vi "HFRR ADV v017 new software.vi"() -> ()   [LabVIEW 2025] (continued)
        n325 = Unbundle By Name("Password 3") -> ("Service Password"=w415:string)
        n326 = call <vilib>:"Trim Whitespace.vi"("string"=w415) -> ("trimmed string"=w413:string)  [unwired: 1 in]
        n327 = Equal?(x=w413, y="Service@123") -> (x = y?=w414:bool)
        n328 = case shown="False" w414 {
          selector: w414 -> [w419 w421]
          frame False {
            n329 = local write "Service Password enable"(w419) -> ()
            n330 = property on="Service Password Log" class="Str"("Visible"=TRUE) -> ()  [unwired: 2 in, 2 out]
            n331 = property on="Tab Control 5" class="TabCtl (strict)"("Tabs Visible?"=TRUE ("Page Labels Display Visible?")) -> ()  [unwired: 2 in, 2 out]
          }
          frame True {
            n332 = property on="Service Password Log" class="Str"("Visible"=FALSE) -> ()  [unwired: 2 in, 2 out]
            "Service Password enable" <- w421
          }
        }
      }
      event "Sign In": Value Change {
        w423 = FALSE ("Visible")
        n333 = event-data() -> ()  [unwired: 1 in, 6 out]
        n334 = property on="About" class="Clust (strict)"("Visible"=w423) -> ()  [unwired: 2 in, 2 out]
        n335 = property on="Password 3" class="Clust (strict)"("Visible"=w423) -> ()  [unwired: 2 in, 2 out]
        n336 = property on="Service Password Log" class="Str"("Visible"=FALSE) -> ()  [unwired: 2 in, 2 out]
      }
      event "Info": Value Change {
        n337 = event-data() -> ()  [unwired: 1 in, 6 out]
        n338 = local read "Info"() -> (w425:bool)
        n339 = case shown="False" w425 {
          frame False {
            n340 = property on="About" class="Clust (strict)"("Visible"=FALSE) -> ()  [unwired: 2 in, 2 out]
          }
          frame True {
            n341 = property on="About" class="Clust (strict)"("Visible"=TRUE) -> ()  [unwired: 2 in, 2 out]
          }
        }
      }
      event "Calibration": Value Change {
        n342 = event-data() -> ()  [unwired: 1 in, 6 out]
        n343 = local read "Calibration"() -> (w429:bool)
        n344 = case shown="False" w429 {
          frame False {
            n345 = property on="Calibration 2" class="TabCtl (strict)"("Visible"=FALSE) -> ()  [unwired: 2 in, 2 out]
            n346 = local write "Cal Password"("" ("Cal Password")) -> ()
          }
          frame True {
            n347 = property on="Calibration 2" class="TabCtl (strict)"("Visible"=TRUE) -> ()  [unwired: 2 in, 2 out]
            n348 = local write "Cal Password"("" ("Cal Password")) -> ()
          }
        }
        n349 = property on="Wrong Password" class="Str"("Visible"=FALSE) -> ()  [unwired: 2 in, 2 out]
      }
      event "Cal Password": Value Change {
        n350 = event-data() -> ()  [unwired: 1 in, 6 out]
        n351 = local read "Cal Password"() -> (w437:string)
        n352 = call <vilib>:"Trim Whitespace.vi"("string"=w437) -> ("trimmed string"=w436:string)  [unwired: 1 in]
        n353 = Equal?(x=w436, y="Cal@321") -> (x = y?=w434:bool)
        n354 = case shown="True" w434 {
          frame False {
            n355 = property on="Wrong Password" class="Str"("Visible"=TRUE) -> ()  [unwired: 2 in, 2 out]
          }
          frame True {
            n356 = property on="Wrong Password" class="Str"("Visible"=FALSE) -> ()  [unwired: 2 in, 2 out]
            n357 = local write "Main Tab"(T2."About" ("Main Tab")) -> ()
            n358 = local write "Cal Password"("" ("Cal Password")) -> ()
            n359 = local write "Main Dashboard Buttons"(T1."About" ("Main Dashboard Buttons")) -> ()
            n360 = local write "Tab Control 5"(T12."Temperature Calibration" ("Tab Control 5")) -> ()
            n361 = property on="Calibration 2" class="TabCtl (strict)"("Visible"=FALSE) -> ()  [unwired: 2 in, 2 out]
            n362 = property on="Tab Control 5" class="TabCtl (strict)"("Tabs Visible?"=FALSE ("Page Labels Display Visible?")) -> ()  [unwired: 2 in, 2 out]
            n363 = local write "Calibration"(FALSE ("Calibration")) -> ()
          }
        }
      }
      event "Calibration Selection": Value Change {
        n364 = event-data() -> ()  [unwired: 1 in, 6 out]
        n365 = local read "Calibration Selection"() -> (w448:T8)
        n366 = case shown="\"Stroke Calibration\"" w448 {
          tunnel: [T7."Stroke" ("Main Calibration Tab") T7."Friction" ("Main Calibration Tab") T7."Main" ("Main Calibration Tab") T7."Temperature" ("Main Calibration Tab")] -> w447
          frame "Stroke Calibration" {
          }
          frame "Friction Force Calibration" {
          }
          frame Default {
          }
          frame "Temperature Calibration" {
          }
        }
        n367 = local write "Main Calibration Tab"(w447) -> ()
      }
      event "Back Stroke": Value Change {
        n368 = event-data() -> ()  [unwired: 1 in, 6 out]
        n369 = local write "Main Stroke Tab"(T9."Step 1" ("Main Stroke Tab")) -> ()
        n370 = local write "Main Calibration Tab"(T7."Main" ("Main Calibration Tab")) -> ()
        n371 = local write "Back Stroke"(FALSE ("Back Stroke")) -> ()
      }
      event "Step 2 Back": Value Change {
        n372 = event-data() -> ()  [unwired: 1 in, 6 out]
        n373 = local write "Main Stroke Tab"(T9."Step 1" ("Main Stroke Tab")) -> ()
        n374 = local write "Step 2 Back"(FALSE ("Back Stroke")) -> ()
      }
      event "Step 3 Back": Value Change {
        n375 = event-data() -> ()  [unwired: 1 in, 6 out]
        n376 = local write "Main Stroke Tab"(T9."Step 2" ("Main Stroke Tab")) -> ()
        n377 = local write "Step 3 Back"(FALSE ("Back Stroke")) -> ()
      }
      event "Step 4 Back": Value Change {
        n378 = event-data() -> ()  [unwired: 1 in, 6 out]
        n379 = local write "Main Stroke Tab"(T9."Step 3" ("Main Stroke Tab")) -> ()
        n380 = local write "Step 4 Back"(FALSE ("Back Stroke")) -> ()
      }
      event "Step 5 Back": Value Change {
        n381 = event-data() -> ()  [unwired: 1 in, 6 out]
        n382 = local write "Main Stroke Tab"(T9."Step 4" ("Main Stroke Tab")) -> ()
        n383 = local write "Step 5 Back"(FALSE ("Back Stroke")) -> ()
      }
      event "Step 6 Back": Value Change {
        n384 = event-data() -> ()  [unwired: 1 in, 6 out]
        n385 = local write "Main Stroke Tab"(T9."Step 5" ("Main Stroke Tab")) -> ()
        n386 = local write "Step 6 Back"(FALSE ("Back Stroke")) -> ()
      }
      event "Back Stroke step 7": Value Change {
        n387 = event-data() -> ()  [unwired: 1 in, 6 out]
        n388 = local write "Main Stroke Tab"(T9."Step 6" ("Main Stroke Tab")) -> ()
        n389 = local write "Back Stroke step 7"(FALSE ("Back Stroke")) -> ()
      }
      event "Back Stroke step 8": Value Change {
        n390 = event-data() -> ()  [unwired: 1 in, 6 out]
        n391 = local write "Main Stroke Tab"(T9."Step 7" ("Main Stroke Tab")) -> ()
        n392 = local write "Back Stroke step 8"(FALSE ("Back Stroke")) -> ()
      }
      event "Back Stroke 8": Value Change {
        n393 = event-data() -> ()  [unwired: 1 in, 6 out]
        n394 = local write "MOVE CARRIAGE TO"(0.2 ("MOVE CARRIAGE TO")) -> ()
        n395 = local write "Main Stroke Tab"(T9."Step 1" ("Main Stroke Tab")) -> ()
        n396 = local write "Back Stroke 8"(FALSE ("Back Stroke 8")) -> ()
      }
      event "Continue Stroke": Value Change {
        n397 = event-data() -> ()  [unwired: 1 in, 6 out]
        n398 = local write "Main Stroke Tab"(T9."Step 2" ("Main Stroke Tab")) -> ()
        n399 = local write "Continue Stroke"(FALSE ("Continue Stroke")) -> ()
      }
      event "Continue Stroke step 2": Value Change {
        n400 = event-data() -> ()  [unwired: 1 in, 6 out]
        n401 = local write "Main Stroke Tab"(T9."Step 3" ("Main Stroke Tab")) -> ()
        n402 = local write "Continue Stroke step 2"(FALSE ("Continue Stroke")) -> ()
      }
      event "Continue Stroke step 3": Value Change {
        n403 = event-data() -> ()  [unwired: 1 in, 6 out]
        n404 = local write "Main Stroke Tab"(T9."Step 4" ("Main Stroke Tab")) -> ()
        n405 = local write "Continue Stroke step 3"(FALSE ("Continue Stroke")) -> ()
      }
      event "Continue Stroke step 4": Value Change {
        n406 = event-data() -> ()  [unwired: 1 in, 6 out]
        n407 = local write "Main Stroke Tab"(T9."Step 5" ("Main Stroke Tab")) -> ()
        n408 = local write "Continue Stroke step 4"(FALSE ("Continue Stroke")) -> ()
      }
      event "Continue Stroke step 5": Value Change {
        n409 = event-data() -> ()  [unwired: 1 in, 6 out]
        n410 = local write "Main Stroke Tab"(T9."Step 6" ("Main Stroke Tab")) -> ()
        n411 = local write "Continue Stroke step 5"(FALSE ("Continue Stroke")) -> ()
      }
      event "Continue Stroke step 6": Value Change {
        n412 = event-data() -> ()  [unwired: 1 in, 6 out]
        n413 = local write "Main Stroke Tab"(T9."Step 7" ("Main Stroke Tab")) -> ()
        n414 = local write "Continue Stroke step 6"(FALSE ("Continue Stroke")) -> ()
      }
      event "Continue Stroke step 7": Value Change {
        w487 = FALSE ("0.2mm")
        n415 = event-data() -> ()  [unwired: 1 in, 6 out]
        n416 = local write "0.4 mm"(w487) -> ()
        n417 = local write "0.6 mm"(w487) -> ()
        n418 = local write "1.0 mm"(w487) -> ()
        n419 = local write "1.2 mm"(w487) -> ()
        n420 = local write "0.2 2"(w487) -> ()
        n421 = local write "0.4 2"(w487) -> ()
        n422 = local write "0.6 2"(w487) -> ()
        n423 = local write "0.8 2"(w487) -> ()
        n424 = local write "1.0 2"(w487) -> ()
        n425 = local write "1.2"(w487) -> ()
        n426 = local write "0.2mm"(w487) -> ()
        n427 = local write "0.8mm"(w487) -> ()
        n428 = local write "Main Stroke Tab"(T9."Step 8" ("Main Stroke Tab")) -> ()
        n429 = local write "Continue Stroke step 7"(FALSE ("Continue Stroke")) -> ()
        n430 = local write "Stroke Test Complete"(T10."Test Progress" ("Stroke Test Complete")) -> ()
        "Position Measurment Temp" <- 0.0 ("Position Measurment Temp")
        "Calibration Tare" <- TRUE ("Calibration Tare")
        "MOVE CARRIAGE TO" <- 0.2 ("MOVE CARRIAGE TO")
      }
      event "Continue Stroke step 8": Value Change {
        n431 = event-data() -> ()  [unwired: 1 in, 6 out]
        n432 = local read "LVDT STROKE  Calibration"() -> (w492:dbl)
        n433 = local read "Position Measurment Temp"() -> (w493:dbl)
        n434 = case shown="4" w493 {
          selector: w493 -> [w498 w503 w508 w513 w518 w522 w525 w526]
          tunnel: w492 -> [w494 w499 w504 w509 w514 w519 _ _]
          frame 0, Default {
            w496 = TRUE ("0.2mm")
            n435 = Increment(x=w498) -> (x+1=w497:i32)
            n436 = local write "Position Measurment Temp"(w497) -> ()
            n437 = local write "0.2mm"(w496) -> ()
            n438 = local write "0.2 2"(w496) -> ()
            n439 = local write "MOVE CARRIAGE TO"(0.4 ("MOVE CARRIAGE TO")) -> ()
            "Calibration 0.2" <- w494
          }
          frame 1 {
            w501 = TRUE ("0.4 mm")
            n440 = Increment(x=w503) -> (x+1=w502:i32)
            n441 = local write "Calibration 0.4"(w499) -> ()
            n442 = local write "Position Measurment Temp"(w502) -> ()
            n443 = local write "0.4 mm"(w501) -> ()
            n444 = local write "MOVE CARRIAGE TO"(0.6 ("MOVE CARRIAGE TO")) -> ()
            n445 = local write "0.4 2"(w501) -> ()
          }
          frame 2 {
            w506 = TRUE ("0.6 mm")
            n446 = Increment(x=w508) -> (x+1=w507:i32)
            n447 = local write "Calibration 0.6"(w504) -> ()
            n448 = local write "Position Measurment Temp"(w507) -> ()
            n449 = local write "0.6 2"(w506) -> ()
            n450 = local write "0.6 mm"(w506) -> ()
            n451 = local write "MOVE CARRIAGE TO"(0.8 ("MOVE CARRIAGE TO")) -> ()
          }
          frame 3 {
            w510 = TRUE ("0.6 mm")
            n452 = Increment(x=w513) -> (x+1=w512:i32)
            n453 = local write "Position Measurment Temp"(w512) -> ()
            n454 = local write "MOVE CARRIAGE TO"(1.0 ("MOVE CARRIAGE TO")) -> ()
            n455 = local write "0.8mm"(w510) -> ()
            n456 = local write "0.8 2"(w510) -> ()
            "Calibration 0.8" <- w509
          }
          frame 4 {
            w515 = TRUE ("0.6 mm")
            n457 = Increment(x=w518) -> (x+1=w517:i32)
            n458 = local write "Position Measurment Temp"(w517) -> ()
            n459 = local write "MOVE CARRIAGE TO"(1.2 ("MOVE CARRIAGE TO")) -> ()
            n460 = local write "1.0 mm"(w515) -> ()
            n461 = local write "1.0 2"(w515) -> ()
            "Calibration 1.0" <- w514
          }
          frame 5 {
            w520 = TRUE ("0.6 mm")
            n462 = Increment(x=w522) -> (x+1=w521:i32)
            n463 = local write "Position Measurment Temp"(w521) -> ()
            n464 = local write "1.2 mm"(w520) -> ()
            n465 = local write "1.2"(w520) -> ()
            "Calibration 1.2" <- w519
          }
          frame 6 {
            n466 = Increment(x=w525) -> (x+1=w524:i32)
            n467 = local write "Position Measurment Temp"(w524) -> ()
            n468 = local write "Stroke Test Complete"(T10."Stroke Points Completed" ("Stroke Test Complete")) -> ()
          }
          frame 7 {
            n469 = stacked-sequence {
              tunnel: w526 -> [w527 _ _]
              frame #0 {
                n470 = Increment(x=w527) -> (x+1=w528:i32)
                n471 = local write "Main Stroke Tab"(T9."Step 9" ("Main Stroke Tab")) -> ()
                n472 = local write "Position Measurment Temp"(w528) -> ()
                n473 = Insert Into Array(array=dbl[] [], new element #1=0.2 ("new element/subarray"), new element #2=0.4 ("new element/subarray"), new element #3=0.6 ("new element/subarray"), new element #4=0.8 ("new element/subarray"), new element #5=1.0 ("new element/subarray"), new element #6=1.2 ("new element/subarray")) -> (→"1D stroke":dbl[])  [unwired: 1 in]
                n474 = local read "Calibration 0.2"() -> (w535:dbl)
                n475 = local read "Calibration 0.4"() -> (w534:dbl)
                n476 = local read "Calibration 0.6"() -> (w533:dbl)
                n477 = local read "Calibration 0.8"() -> (w532:dbl)
                n478 = local read "Calibration 1.0"() -> (w531:dbl)
                n479 = local read "Calibration 1.2"() -> (w530:dbl)
                n480 = Insert Into Array(array=dbl[] [], new element #1=w535, new element #2=w534, new element #3=w533, new element #4=w532, new element #5=w531, new element #6=w530) -> (→"Calibrated Voltage Value":dbl[])  [unwired: 1 in]
              }
              frame #1 {
                n481 = local read "Calibrated Voltage Value"() -> (w547:dbl[])
                n482 = local read "1D stroke"() -> (w548:dbl[])
                n483 = for {
                  tunnel: [w551] -> w546 mode=indexing
                  tunnel: w548 -> [w550] mode=indexing
                  tunnel: w547 -> [w549] mode=indexing
                  n484 = formula code="if (stroke == 0.2) {\n    status = (voltage >= 0.0961 && voltage <= 0.4961) ? 1 : 0;\n} else if (stroke == 0.4) {\n    status = (voltage >= 0.3425 && voltage <= 0.7425) ? 1 : 0;\n} else if (stroke == 0.6) {\n    status = (voltage >= 0.5370 && voltage <= 0.9370) ? 1 : 0;\n} else if (stroke == 0.8) {\n    status = (voltage >= 0.6640 && voltage <= 1.0640) ? 1 : 0;\n} else if (stroke == 1.0) {\n    status = (voltage >= 0.9000 && voltage <= 1.1000) ? 1 : 0;\n} else if (stroke == 1.2) {\n    status = (voltage >= 0.9278 && voltage <= 1.3278) ? 1 : 0;\n} else {\n    status = 0; // Fails if an invalid stroke value is supplied\n}"("stroke"=w550, "voltage"=w549) -> ("status"=w551:dbl)
                }
                "Status" <- w546
              }
              frame #2 {
                w558 = 1.0
                n485 = local read "Status"() -> (w565:dbl[])
                n486 = Index Array(array=w565) -> (element #1=w564:dbl, element #2=w563:dbl, element #3=w562:dbl, element #4=w561:dbl, element #5=w560:dbl, element #6=w559:dbl)  [unwired: 6 in]
                n487 = Equal?(x=w563, y=w558) -> (x = y?=w556:bool)
                n488 = Equal?(x=w562, y=w558) -> (x = y?=w555:bool)
                n489 = Equal?(x=w561, y=w558) -> (x = y?=w554:bool)
                n490 = Equal?(x=w560, y=w558) -> (x = y?=w553:bool)
                n491 = Equal?(x=w559, y=w558) -> (x = y?=w552:bool)
                n492 = Equal?(x=w564, y=w558) -> (x = y?=w557:bool)
                n493 = case shown="True" w557 {
                  selector: w557 -> [w576 w577]
                  frame True {
                    n494 = local write "Point 1 - 0.2 mm"(w576) -> ()
                    n495 = property on="Point 1 - 0.2 mm" class="Bool"("Caption.Visible"=w576) -> ()  [unwired: 2 in, 2 out]
                  }
                  frame False {
                    n496 = local write "Point 1 - 0.2 mm"(w577) -> ()
                    n497 = property on="Point 1 - 0.2 mm" class="Bool"("Caption.Visible"=w577) -> ()  [unwired: 2 in, 2 out]
                  }
                }
                n498 = case shown="True" w556 {
                  selector: w556 -> [w574 w575]
                  frame True {
                    n499 = local write "Point 2 - 0.4 mm"(w574) -> ()
                    n500 = property on="Point 2 - 0.4 mm" class="Bool"("Caption.Visible"=w574) -> ()  [unwired: 2 in, 2 out]
                  }
                  frame False {
                    n501 = local write "Point 2 - 0.4 mm"(w575) -> ()
                    n502 = property on="Point 2 - 0.4 mm" class="Bool"("Caption.Visible"=w575) -> ()  [unwired: 2 in, 2 out]
                  }
                }
                n503 = case shown="True" w553 {
                  selector: w553 -> [w568 w569]
                  frame True {
                    n504 = local write "Point 5 - 1.0 mm"(w568) -> ()
                    n505 = property on="Point 5 - 1.0 mm" class="Bool"("Caption.Visible"=w568) -> ()  [unwired: 2 in, 2 out]
                  }
                  frame False {
                    n506 = local write "Point 5 - 1.0 mm"(w569) -> ()
                    n507 = property on="Point 5 - 1.0 mm" class="Bool"("Caption.Visible"=w569) -> ()  [unwired: 2 in, 2 out]
                  }
                }
                n508 = case shown="True" w555 {
                  selector: w555 -> [w572 w573]
                  frame True {
                    n509 = local write "Point 3 - 0.6 mm"(w572) -> ()
                    n510 = property on="Point 3 - 0.6 mm" class="Bool"("Caption.Visible"=w572) -> ()  [unwired: 2 in, 2 out]
                  }
                  frame False {
                    n511 = local write "Point 3 - 0.6 mm"(w573) -> ()
                    n512 = property on="Point 3 - 0.6 mm" class="Bool"("Caption.Visible"=w573) -> ()  [unwired: 2 in, 2 out]
                  }
                }
                n513 = case shown="True" w554 {
                  selector: w554 -> [w570 w571]
                  frame True {
                    n514 = local write "Point 4 - 0.8 mm"(w570) -> ()
                    n515 = property on="Point 4 - 0.8 mm" class="Bool"("Caption.Visible"=w570) -> ()  [unwired: 2 in, 2 out]
                  }
                  frame False {
                    n516 = local write "Point 4 - 0.8 mm"(w571) -> ()
                    n517 = property on="Point 4 - 0.8 mm" class="Bool"("Caption.Visible"=w571) -> ()  [unwired: 2 in, 2 out]
                  }
                }
                n518 = case shown="True" w552 {
                  selector: w552 -> [w566 w567]
                  frame True {
                    n519 = local write "Point 6 - 1.2 mm"(w566) -> ()
                    n520 = property on="Point 6 - 1.2 mm" class="Bool"("Caption.Visible"=w566) -> ()  [unwired: 2 in, 2 out]
                  }
                  frame False {
                    n521 = local write "Point 6 - 1.2 mm"(w567) -> ()
                    n522 = property on="Point 6 - 1.2 mm" class="Bool"("Caption.Visible"=w567) -> ()  [unwired: 2 in, 2 out]
                  }
                }
              }
            }
          }
        }
      }
      event "TEMPERATURE STEP Back 1", "TEMPERATURE STEP Back air Temp": Value Change {
        n523 = event-data() -> ()  [unwired: 1 in, 6 out]
        n524 = stacked-sequence {
          frame #0 {
            n525 = local write "Main Calibration Tab"(T7."Main" ("Main Calibration Tab")) -> ()
          }
          frame #1 {
            n526 = Wait (ms)(milliseconds to wait=u32 1000) -> ()  [unwired: 1 out]
          }
          frame #2 {
            n527 = local write "Command"("CAL;END" ("Command")) -> ()
          }
          frame #3 {
            n528 = Wait (ms)(milliseconds to wait=u32 2000) -> ()  [unwired: 1 out]
          }
          frame #4 {
            n529 = local write "Command"("CAL;END" ("Command")) -> ()
          }
        }
      }
      event "Temperature Continue Step 1": Value Change {
        n530 = event-data() -> ()  [unwired: 1 in, 6 out]
        n531 = stacked-sequence {
          frame #0 {
            n532 = Wait (ms)(milliseconds to wait=u32 1500) -> ()  [unwired: 1 out]
          }
          frame #1 {
            n533 = local write "Command"("CAL;START" ("Command")) -> ()
          }
          frame #2 {
            n534 = Wait (ms)(milliseconds to wait=u32 1500) -> ()  [unwired: 1 out]
          }
          frame #3 {
            n535 = local write "Command"("CAL;START" ("Command")) -> ()
          }
          frame #4 {
            n536 = Wait (ms)(milliseconds to wait=u32 2000) -> ()  [unwired: 1 out]
          }
          frame #5 {
          }
          frame #6 {
            n537 = Wait (ms)(milliseconds to wait=u32 2000) -> ()  [unwired: 1 out]
          }
          frame #7 {
            # "CAL;A1;<true_T>"
            n538 = local write "Command"("CAL;A1;0" ("Command")) -> ()
          }
          frame #8 {
            n539 = local write "Tab Control 4"(T11."Step 2" ("Tab Control 4")) -> ()
          }
        }
      }
      event "Temperature Continue Step air Step 1": Value Change {
        n540 = event-data() -> ()  [unwired: 1 in, 6 out]
        n541 = stacked-sequence {
          frame #0 {
            n542 = Wait (ms)(milliseconds to wait=u32 1500) -> ()  [unwired: 1 out]
          }
          frame #1 {
            n543 = local write "Command"("CAL;START" ("Command")) -> ()
          }
          frame #2 {
            n544 = local write "Tab Control 4"(T11."Air Step 2" ("Tab Control 4")) -> ()
            n545 = Wait (ms)(milliseconds to wait=u32 1500) -> ()  [unwired: 1 out]
          }
          frame #3 {
            n546 = local write "Command"("CAL;START" ("Command")) -> ()
          }
          frame #4 {
            n547 = Wait (ms)(milliseconds to wait=u32 2000) -> ()  [unwired: 1 out]
          }
          frame #5 {
            # "CAL;A1;<true_T>"
            n548 = local write "Command"("CAL;A2;0" ("Command")) -> ()
          }
          frame #6 {
            n549 = Wait (ms)(milliseconds to wait=u32 2000) -> ()  [unwired: 1 out]
          }
          frame #7 {
            # "CAL;A1;<true_T>"
            n550 = local write "Command"("CAL;A1;0" ("Command")) -> ()
          }
        }
      }
      event "Temperature Selection": Value Change {
        n551 = event-data() -> ()  [unwired: 1 in, 6 out]
        n552 = local read "Temperature Selection"() -> (w600:enum32{"Air Temperature", "Sample Temperature"})
        n553 = case shown="\"Sample Temperature\"" w600 {
          frame "Air Temperature", Default {
            n554 = local write "Tab Control 4"(T11."Air Step 1" ("Tab Control 4")) -> ()
          }
          frame "Sample Temperature" {
            n555 = local write "Tab Control 4"(T11."Step 1" ("Tab Control 4")) -> ()
          }
        }
      }
      event "Temperature Continue Step 2": Value Change {
        n556 = event-data() -> ()  [unwired: 1 in, 6 out]
        n557 = stacked-sequence {
          frame #0 {
            n558 = stacked-sequence {
              frame #0 {
                n559 = Wait (ms)(milliseconds to wait=u32 1500) -> ()  [unwired: 1 out]
              }
              frame #1 {
                # "CAL;A1;<true_T>"
                n560 = local write "Command"("CAL;A1;0" ("Command")) -> ()
              }
              frame #2 {
                n561 = Wait (ms)(milliseconds to wait=u32 1500) -> ()  [unwired: 1 out]
              }
              frame #3 {
                # "CAL;A1;<true_T>"
                n562 = local write "Command"("CAL;A1;0" ("Command")) -> ()
              }
              frame #4 {
              }
            }
          }
          frame #1 {
            n563 = local write "Tab Control 4"(T11."Step 3" ("Tab Control 4")) -> ()
          }
        }
      }
      event "Temperature Continue Step 3": Value Change {
        n564 = event-data() -> ()  [unwired: 1 in, 6 out]
        n565 = stacked-sequence {
          frame #0 {
            n566 = stacked-sequence {
              frame #0 {
                n567 = Wait (ms)(milliseconds to wait=u32 1500) -> ()  [unwired: 1 out]
              }
              frame #1 {
              }
              frame #2 {
              }
              frame #3 {
                # "CAL;A1;<true_T>"
                n568 = local write "Command"("CAL;A1;60" ("Command")) -> ()
              }
              frame #4 {
                n569 = Wait (ms)(milliseconds to wait=u32 2000) -> ()  [unwired: 1 out]
              }
              frame #5 {
                # "CAL;A1;<true_T>"
                n570 = local write "Command"("CAL;A1;60" ("Command")) -> ()
              }
            }
          }
          frame #1 {
            n571 = Wait (ms)(milliseconds to wait=u32 1000) -> ()  [unwired: 1 out]
          }
          frame #2 {
            n572 = local write "Command"("CAL;SAVE" ("Command")) -> ()
          }
          frame #3 {
            n573 = Wait (ms)(milliseconds to wait=u32 1000) -> ()  [unwired: 1 out]
          }
          frame #4 {
            n574 = local write "Command"("CAL;SAVE" ("Command")) -> ()
          }
          frame #5 {
            n575 = Wait (ms)(milliseconds to wait=u32 1000) -> ()  [unwired: 1 out]
          }
          frame #6 {
            # "CAL;END"
            n576 = local write "Command"("CAL;END" ("Command")) -> ()
          }
          frame #7 {
            n577 = Wait (ms)(milliseconds to wait=u32 1000) -> ()  [unwired: 1 out]
          }
          frame #8 {
            # "CAL;END"
            n578 = local write "Command"("CAL;END" ("Command")) -> ()
          }
          frame #9 {
            n579 = local write "Main Calibration Tab"(T7."Temperature" ("Main Calibration Tab")) -> ()
            n580 = local write "Tab Control 4"(T11."Main" ("Tab Control 4")) -> ()
          }
        }
      }
      event "Back Stroke step main temperature": Value Change {
        n581 = event-data() -> ()  [unwired: 1 in, 6 out]
        n582 = stacked-sequence {
          frame #0 {
            n583 = Wait (ms)(milliseconds to wait=u32 1000) -> ()  [unwired: 1 out]
          }
          frame #1 {
            # "CAL;END"
            n584 = local write "Command"("CAL;END" ("Command")) -> ()
          }
          frame #2 {
            n585 = Wait (ms)(milliseconds to wait=u32 1000) -> ()  [unwired: 1 out]
          }
          frame #3 {
            # "CAL;END"
            n586 = local write "Command"("CAL;END" ("Command")) -> ()
          }
          frame #4 {
            n587 = local write "Main Calibration Tab"(T7."Temperature" ("Main Calibration Tab")) -> ()
            n588 = local write "Tab Control 4"(T11."Main" ("Tab Control 4")) -> ()
          }
        }
      }
      event "Quit": Value Change {
        n589 = event-data() -> ()  [unwired: 1 in, 6 out]
      }
    }
    n590 = Wait (ms)(milliseconds to wait=u32 100) -> ()  [unwired: 1 out]
  }
  n591 = while {
    stop <- w632 stop-if-true
    n592 = local read "Ambient Temperature"() -> (w630:dbl)
    n593 = local read "Sample Temperature"() -> (w629:dbl)
    n594 = local write "Temperature — Live (Set A: 60 °C)"(w629) -> ()
    n595 = local write "Temperature — Live (Set A: 60 °C)"(w629) -> ()
    n596 = local write "Temperature — Live (Set A: 0 °C)"(w630) -> ()
    n597 = local write "Sensor value"(w630) -> ()
    n598 = local write "Sensor value"(w629) -> ()
    n599 = local write "Temperature — Live (Set A: 60 °C)"(w630) -> ()
    n600 = local write "Sensor value"(w629) -> ()
    n601 = local write "Sensor value"(w630) -> ()
    n602 = Wait (ms)(milliseconds to wait=u32 200) -> ()  [unwired: 1 out]
    n603 = local read "Quit"() -> (w632:bool)
  }
  n604 = while {
    shift-right: [w634] -> _
    shift-left: "Enum - Selector" -> [w635]
    stop <- w636 stop-if-true
    # "Auto Start Logic Loop"
    n605 = case shown="\"Maintain Stage\"" w635 {
      tunnel: [w639 w645 w672 w704 w734 Auto_Start_enum."Exit" ("Enum - Selector") Auto_Start_enum."Init" ("Enum - Selector")] -> w634
      frame "Init", Default {
        n606 = local read "Auto Start Test"() -> (w638:bool)
        n607 = Select(t=Auto_Start_enum."Humidity & Temperature On" ("Enum - Selector"), s=w638, f=Auto_Start_enum."Init") -> (s? t:f=w639:T15)
      }
      frame "Humidity & Temperature On" {
        n608 = stacked-sequence {
          tunnel: [_ _ _ _ _ _ Auto_Start_enum."Reach point" ("Enum - Selector")] -> w642
          frame #0 {
            w647 = T19."Disabled and Grayed Out" ("Disabled")
            w648 = TRUE ("Heater Button")
            n609 = property on="Humidity" class="Bool (strict)"("DisabledEnum"=w647) -> ()  [unwired: 2 in, 2 out]
            n610 = property on="Heater Button" class="Bool (strict)"("DisabledEnum"=w647) -> ()  [unwired: 2 in, 2 out]
            n611 = local write "Heater Button"(w648) -> ()
            n612 = local write "Humidity"(w648) -> ()
            n613 = property on="Heater Button" class="Bool (strict)"("Val(Sgnl)"=TRUE ("Value (Signaling)")) -> ()  [unwired: 2 in, 2 out]
          }
          frame #1 {
            n614 = Wait (ms)(milliseconds to wait=u32 3000) -> ()  [unwired: 1 out]
          }
          frame #2 {
            n615 = local read "Set Temp"() -> (w654:dbl)
            n616 = Number To Fractional String(number=w654, precision (6)=i16 2) -> (F-format string=w651:string)  [unwired: 2 in]
            n617 = Concatenate Strings("ST;" ("Command"), w651) -> (w652:string)
            n618 = local write "Command"(w652) -> ()
          }
          frame #3 {
            n619 = Wait (ms)(milliseconds to wait=u32 1500) -> ()  [unwired: 1 out]
          }
          frame #4 {
            (unwired) i16 2 ("precision (6)")
            n620 = local read "Set Rh"() -> (w657:dbl)
            n621 = Number To Fractional String(number=w657) -> (F-format string=w660:string)  [unwired: 3 in]
            n622 = local read "WriteHumidity"() -> (w658:string[])
            n623 = Concatenate Strings("M;" ("new element/subarray"), w660) -> (w661:string)
            n624 = local write "Command"("HE;1" ("Command")) -> ()
            n625 = Insert Into Array(array=w658, new element=w661) -> (w659:string[])  [unwired: 1 in]
            n626 = local write "WriteHumidity"(w659) -> ()
          }
          frame #5 {
            n627 = Wait (ms)(milliseconds to wait=u32 1500) -> ()  [unwired: 1 out]
          }
          frame #6 {
            w664 = TRUE ("Reach point temp")
            n628 = local write "Reach point Humidity"(w664) -> ()
            n629 = local write "Reach point temp"(w664) -> ()
          }
        }
        n630 = local read "Auto Start Test"() -> (w644:bool)
        n631 = Not(x=w644) -> (.not. x?=w643:bool)
        n632 = Select(t=Auto_Start_enum."close", s=w643, f=w642) -> (s? t:f=w645:T15)
      }
      frame "Reach point" {
        w673 = TRUE ("PAUSE")
        w681 = 1.0 ("y")
        w684 = 1.0 ("y")
        n633 = local read "Set Temp"() -> (w666:dbl)
        n634 = local read "Set Humidity:"() -> (w680:dbl)
        n635 = local read "Humidity ( %RH )"() -> (w685:dbl)
        n636 = Add(x=w666, y=w684) -> (x+y=w683:dbl)
        n637 = Subtract(x=w666, y=w684) -> (x-y=w682:dbl)
        n638 = Add(x=w680, y=w681) -> (x+y=w679:dbl)
        n639 = Subtract(x=w680, y=w681) -> (x-y=w678:dbl)
        n640 = local read "TEMP"() -> (w686:dbl)
        n641 = In Range and Coerce(upper limit=w679, x=w685, lower limit=w678) -> (In Range?=w667:bool)  [unwired: 1 out]
        n642 = In Range and Coerce(upper limit=w683, x=w686, lower limit=w682) -> (In Range?=w668:bool)  [unwired: 1 out]
        n643 = case shown="True" w667 {
          frame False {
          }
          frame True {
            n644 = case shown="True" "Reach point Humidity" {
              selector: "Reach point Humidity" -> [_ w692]
              frame False {
              }
              frame True {
                n645 = local read "EVENT LOG"() -> (w689:string)
                n646 = Not(x=w692) -> (.not. x?=w691:bool)
                n647 = local write "Reach point Humidity"(w691) -> ()
                n648 = call "Event Log.vi"("Content"="Target Humidity reached", "EVENT LOG"=w689) -> ("EVENT LOG"=w690:string)  [unwired: 8 in, 1 out]
                n649 = local write "EVENT LOG"(w690) -> ()
              }
            }
          }
        }
        n650 = case shown="True" w668 {
          frame False {
          }
          frame True {
            n651 = case shown="True" "Reach point temp" {
              selector: "Reach point temp" -> [_ w698]
              frame False {
              }
              frame True {
                n652 = local read "EVENT LOG"() -> (w695:string)
                n653 = Not(x=w698) -> (.not. x?=w697:bool)
                n654 = local write "Reach point temp"(w697) -> ()
                n655 = call "Event Log.vi"("Content"="Target Temperature reached", "EVENT LOG"=w695) -> ("EVENT LOG"=w696:string)  [unwired: 8 in, 1 out]
                n656 = local write "EVENT LOG"(w696) -> ()
              }
            }
          }
        }
        n657 = local read "Auto Start Test"() -> (w671:bool)
        n658 = And(x=w668, y=w667) -> (x .and. y?=w677:bool)
        n659 = Select(t=Auto_Start_enum."Maintain Stage" ("Enum - Selector"), s=w677, f=Auto_Start_enum."Reach point" ("Enum - Selector")) -> (s? t:f=w674:T15)
        n660 = Not(x=w671) -> (.not. x?=w670:bool)
        n661 = Select(t=Auto_Start_enum."close", s=w670, f=w674) -> (s? t:f=w672:T15)
        n662 = call "ELAPSED TIMER VI.vi"("RESET"=w673, "PAUSE"=w673) -> ()  [unwired: 7 in, 3 out]
      }
      frame "Maintain Stage" {
        w713 = 2.0 ("y")
        w712 = 1.0 ("y")
        # "Humidity and  temperatures Set Point  have been reached"
        n663 = local read "Set Temp"() -> (w699:dbl)
        n664 = local read "Set Humidity:"() -> (w716:dbl)
        n665 = local read "Humidity ( %RH )"() -> (w719:dbl)
        n666 = Add(x=w699, y=w712) -> (x+y=w718:dbl)
        n667 = Subtract(x=w699, y=w712) -> (x-y=w717:dbl)
        n668 = local read "TEMP"() -> (w720:dbl)
        n669 = Add(x=w716, y=w713) -> (x+y=w715:dbl)
        n670 = Subtract(x=w716, y=w713) -> (x-y=w714:dbl)
        n671 = In Range and Coerce(upper limit=w718, x=w720, lower limit=w717) -> (In Range?=w711:bool)  [unwired: 1 out]
        n672 = In Range and Coerce(upper limit=w715, x=w719, lower limit=w714) -> (In Range?=w710:bool)  [unwired: 1 out]
        n673 = And(x=w711, y=w710) -> (x .and. y?=w709:bool)
        n674 = Not(x=w709) -> (.not. x?=w708:bool)
        n675 = call "ELAPSED TIMER VI.vi"("TARGET"=60.0, "RESET"=w708, "PAUSE"=FALSE) -> ("ELAPSED INDICATION"=w705:bool)  [unwired: 6 in, 2 out]
        n676 = case shown="True" w705 {
          tunnel: w705 -> [_ w723]
          tunnel: [Auto_Start_enum."Maintain Stage" ("Enum - Selector") w722] -> w703
          frame False {
          }
          frame True {
            n677 = stacked-sequence {
              tunnel: w723 -> [_ _ _ _ _]
              tunnel: [_ _ _ _ Auto_Start_enum."Start Stage" ("Enum - Selector")] -> w722
              frame #0 {
                n678 = local read "EVENT LOG"() -> (w725:string)
                n679 = call "Event Log.vi"("Content"="Humidity and temperature set point has stabilized.", "EVENT LOG"=w725) -> ("EVENT LOG"=w726:string)  [unwired: 8 in, 1 out]
                n680 = local write "EVENT LOG"(w726) -> ()
              }
              frame #1 {
                n681 = Wait (ms)(milliseconds to wait=u32 100) -> ()  [unwired: 1 out]
              }
              frame #2 {
                n682 = local read "EVENT LOG"() -> (w729:string)
                n683 = call "Event Log.vi"("Content"="Auto Test Started", "EVENT LOG"=w729) -> ("EVENT LOG"=w730:string)  [unwired: 8 in, 1 out]
                n684 = local write "EVENT LOG"(w730) -> ()
              }
              frame #3 {
                w731 = TRUE ("RUN")
                n685 = local write "RUN"(w731) -> ()
                n686 = property on="Auto Start Temp" class="Bool (strict)"("Val(Sgnl)"=w731) -> ()  [unwired: 2 in, 2 out]
                "Auto Start Temp" <- w731
              }
              frame #4 {
              }
            }
          }
        }
        n687 = local read "Auto Start Test"() -> (w702:bool)
        n688 = Not(x=w702) -> (.not. x?=w701:bool)
        n689 = Select(t=Auto_Start_enum."close", s=w701, f=w703) -> (s? t:f=w704:T15)
      }
      frame "Start Stage" {
        w733 = TRUE ("PAUSE")
        n690 = local read "Auto Start Test"() -> (w738:bool)
        n691 = Not(x=w738) -> (.not. x?=w737:bool)
        n692 = Select(t=Auto_Start_enum."close" ("Enum - Selector"), s=w737, f=Auto_Start_enum."Start Stage" ("Enum - Selector")) -> (s? t:f=w734:T15)
        n693 = call "ELAPSED TIMER VI.vi"("RESET"=w733, "PAUSE"=w733) -> ()  [unwired: 7 in, 3 out]
      }
      frame "close" {
        w740 = FALSE ("Heater Button")
        n694 = local write "RUN"(w740) -> ()
        n695 = local write "Heater Button"(w740) -> ()
        n696 = local write "Humidity"(w740) -> ()
        n697 = local write "Auto Start Test"(w740) -> ()
        n698 = property on="Heater Button" class="Bool (strict)"("Val(Sgnl)"=FALSE ("Value (Signaling)")) -> ()  [unwired: 2 in, 2 out]
      }
      frame "Exit" {
      }
    }
    n699 = Wait (ms)(milliseconds to wait=u32 100) -> ()  [unwired: 1 out]
    n700 = local read "Quit"() -> (w636:bool)
  }
  n701 = property on="Service Password Log" class="Str"("Visible"=w15) -> ()  [unwired: 2 in, 2 out]
  n702 = property on="Password 3" class="Clust (strict)"("Visible"=w15) -> ()  [unwired: 2 in, 2 out]
  n703 = while {
    stop <- w769 stop-if-true
    w752 = errorcluster {"status"=FALSE, "code"=0, "source"=""} ("error in (no error) 3")
    # "this loop is for manual report generation"
    n704 = local read "Confirm Measrurement"() -> (w751:bool)
    n705 = case shown="True" w751 {
      selector: w751 -> [_ w859]
      tunnel: errorcluster {"status"=FALSE, "code"=0, "source"=""} ("error in (no error) 3") -> [_ w860]
      tunnel: [_ w858] -> _
      frame False {
      }
      frame True {
        n706 = stacked-sequence {
          tunnel: w860 -> [_ w893 _]
          tunnel: w859 -> [_ _ w1000]
          tunnel: [_ w881 _] -> w858
          frame #0 {
            n707 = String To Path(string="C:\\LAB-IQ\\Image Calibrate v01.dcf") -> (path=w863:path)
            n708 = Open/Create/Replace File ("Open File")(file path (use dialog)=w863) -> (refnum out=w864:refnum<file>)  [unwired: 5 in, 2 out]
            n709 = for {
              N: 4 -> [_]
              tunnel: w864 -> [w870]
              i -> [w866]
              n710 = Read from Text File ("Read File")(file (use dialog)=w870) -> (text=w871:string)  [unwired: 3 in, 3 out]
              n711 = String Subset(string=w871, offset (0)=6, length (rest)=10 ("length (rest)")) -> (substring=w867:string)
              n712 = Fract/Exp String To Number(string=w867) -> (number=w865:dbl)  [unwired: 3 in, 1 out]
              n713 = case shown="3" w866 {
                tunnel: w865 -> [w872 w873 _ w874 _]
                frame 0 {
                  n714 = local write "5x Gain"(w872) -> ()
                }
                frame 1 {
                  n715 = local write "10x Gain"(w873) -> ()
                }
                frame 2 {
                }
                frame 3 {
                  n716 = local write "100x gain"(w874) -> ()
                }
                frame 4, Default {
                }
              }
            }
          }
          frame #1 {
            n717 = local read "TEST STANDARD"() -> (w876:T3)
            n718 = case shown="\"ISO 12156\"" w876 {
              tunnel: ["ASTM D6079" "ISO 12156"] -> w875
              frame "ASTM D6079", Default {
              }
              frame "ISO 12156" {
              }
            }
            n719 = call "IMAGE ANALYSIS.vi"("Enum"=POST_ANALYSIS_ENUM."GET MEASUREMENTS", "error in"=w893) -> ("error out"=w900:errorcluster)  [unwired: 8 in, 1 out]
            n720 = local read "Magnification :"() -> (w886:string)
            n721 = call "Stall Data Flow.vim"("value in"=w900, "milliseconds to wait"=u32 1000) -> ("value out"=w899:errorcluster)  [unwired: 1 out]
            n722 = local read "Test File List :"() -> (w897:string)
            n723 = case shown="\"10x\"" w886 {
              tunnel: [w936 w937] -> w884
              frame "5x", Default {
                n724 = local read "5x Gain"() -> (w936:dbl)
              }
              frame "10x" {
                # "5x"
                n725 = local read "10x Gain"() -> (w937:dbl)
              }
            }
            n726 = call "IMAGE ANALYSIS.vi"("Enum"=POST_ANALYSIS_ENUM."READ", "error in"=w899) -> ("error out"=w896:errorcluster, "data out"=w887:string)  [unwired: 8 in]
            n727 = Match Pattern(string=w887, regular expression="\"type\": ") -> (after substring=w891:string)  [unwired: 1 in, 3 out]
            n728 = call "IMAGE PATH CREATION PY.vi"("error in (no error)"=w896, "File Name :"=w897) -> ("error out"=w895:errorcluster, "File Path"=w883:path, "File Path String:"=w878:string)  [unwired: 7 in]
            n729 = Match Pattern(string=w891, regular expression=",") -> (before substring=w877:string)  [unwired: 1 in, 3 out]
            n730 = local read "Calibration Tab"() -> (w880:enum32{"Measrument", "Calibrate"})
            n731 = call "Stall Data Flow.vim"("value in"=w895, "milliseconds to wait"=u32 250) -> ("value out"=w879:errorcluster)  [unwired: 1 out]
            n732 = Equal?(x=w877, y="\"rectangle\"") -> (x = y?=w888:bool)
            n733 = case shown="False" w888 {
              tunnel: w887 -> [w942 w997]
              tunnel: w884 -> [_ w988]
              tunnel: cluster{"major":dbl, "minor":dbl, "average":dbl} {"major"=0.0, "minor"=0.0, "average"=0.0} -> [w940 w984]
              tunnel: [w939 w981] -> w882
              tunnel: w877 -> [w941 _]
              tunnel: w884 -> [w938 _]
              frame False {
                n734 = Equal?(x=w941, y="\"line\"") -> (x = y?=w943:bool)
                n735 = case shown="True" w943 {
                  tunnel: w942 -> [_ w958]
                  tunnel: w940 -> [w945 w957]
                  tunnel: [w945 w955] -> w939
                  tunnel: w938 -> [_ w954]
                  frame False {
                  }
                  frame True {
                    w953 = 0.0 ("Major Axis")
                    n736 = Match Pattern(string=w958, regular expression="\"length_px\":") -> (after substring=w956:string)  [unwired: 1 in, 3 out]
                    n737 = property on="Major Axis" class="DigNum (strict)"("Caption.Text"="") -> ()  [unwired: 2 in, 2 out]
                    n738 = property on="Minor Axis" class="DigNum (strict)"("Caption.Text"="") -> ()  [unwired: 2 in, 2 out]
                    n739 = property on="Average" class="DigNum (strict)"("Caption.Text"="Line") -> ()  [unwired: 2 in, 2 out]
                    n740 = Fract/Exp String To Number(string=w956, default (0 dbl)=0.0 ("default (0 DBL)")) -> (number=w952:dbl)  [unwired: 2 in, 1 out]
                    "Pixel Value" <- w952
                    n741 = Multiply(x=w952, y=w954) -> (x*y=w965:dbl)
                    n742 = Multiply(x=w965, y=1000.0) -> (x*y=w948:dbl)
                    n743 = Divide(x=w948, y=1000.0) -> (x/y=w951:dbl)
                    n744 = local write "Measurment (mm)"(w951) -> ()
                    n745 = Bundle By Name(cluster=w957, "average"=w948) -> (w955:cluster{"major":dbl, "minor":dbl, "average":dbl})
                    n746 = Number To Fractional String(number=w948, precision (6)=i16 1) -> (F-format string=w947:string)  [unwired: 2 in]
                    n747 = local write "Minor Axis"(w953) -> ()
                    n748 = local write "Major Axis"(w953) -> ()
                    n749 = Fract/Exp String To Number(string=w947) -> (number=w946:dbl)  [unwired: 3 in, 1 out]
                    n750 = local write "Average"(w946) -> ()
                  }
                }
              }
              frame True {
                w985 = 1000.0 ("y")
                w991 = 0.0 ("default (0 DBL)")
                n751 = Match Pattern(string=w997, regular expression=" \"width_px\":") -> (after substring=w995:string)  [unwired: 1 in, 3 out]
                n752 = Match Pattern(string=w995, regular expression="\"height_px\":") -> (before substring=w993:string, after substring=w992:string)  [unwired: 1 in, 2 out]
                n753 = Fract/Exp String To Number(string=w993, default (0 dbl)=w991) -> (number=w990:dbl)  [unwired: 2 in, 1 out]
                n754 = Fract/Exp String To Number(string=w992, default (0 dbl)=w991) -> (number=w989:dbl)  [unwired: 2 in, 1 out]
                n755 = Multiply(x=w990, y=w988) -> (x*y=w987:dbl)
                n756 = Multiply(x=w989, y=w988) -> (x*y=w986:dbl)
                n757 = Multiply(x=w987, y=w985) -> (x*y=w971:dbl)
                n758 = Multiply(x=w986, y=w985) -> (x*y=w969:dbl)
                n759 = Add(x=w971, y=w969) -> (x+y=w983:dbl)
                n760 = property on="Major Axis" class="DigNum (strict)"("Caption.Text"="Major Axis") -> ()  [unwired: 2 in, 2 out]
                n761 = property on="Minor Axis" class="DigNum (strict)"("Caption.Text"="Minor Axis") -> ()  [unwired: 2 in, 2 out]
                n762 = property on="Average" class="DigNum (strict)"("Caption.Text"="Average") -> ()  [unwired: 2 in, 2 out]
                n763 = Divide(x=w983, y=2.0) -> (x/y=w967:dbl)
                n764 = Bundle By Name(cluster=w984, "major"=w971, "minor"=w969, "average"=w967) -> (w981:cluster{"major":dbl, "minor":dbl, "average":dbl})
                n765 = Number To Fractional String(number=w969, precision (6)=i16 1) -> (F-format string=w976:string)  [unwired: 2 in]
                n766 = Number To Fractional String(number=w967, precision (6)=i16 1) -> (F-format string=w977:string)  [unwired: 2 in]
                n767 = Number To Fractional String(number=w971, precision (6)=i16 1) -> (F-format string=w975:string)  [unwired: 2 in]
                n768 = Fract/Exp String To Number(string=w976) -> (number=w968:dbl)  [unwired: 3 in, 1 out]
                n769 = Fract/Exp String To Number(string=w977) -> (number=w966:dbl)  [unwired: 3 in, 1 out]
                n770 = Fract/Exp String To Number(string=w975) -> (number=w970:dbl)  [unwired: 3 in, 1 out]
                n771 = local write "Major Axis"(w970) -> ()
                n772 = local write "Average"(w966) -> ()
                n773 = local write "Minor Axis"(w968) -> ()
              }
            }
            n774 = case shown="\"Measrument\", Default" w880 {
              tunnel: w883 -> [w910 _]
              tunnel: w882 -> [w909 _]
              tunnel: [w906 w935] -> w881
              tunnel: w879 -> [w908 w935]
              tunnel: w878 -> [w907 _]
              tunnel: w875 -> [w905 _]
              frame "Measrument", Default {
                n775 = stacked-sequence {
                  tunnel: w910 -> [w928 _]
                  tunnel: w909 -> [w926 _]
                  tunnel: w908 -> [w924 _]
                  tunnel: w907 -> [w923 _]
                  tunnel: [w918 _] -> w906
                  tunnel: w905 -> [w911 _]
                  frame #0 {
                    n776 = call "IMAGE ANALYSIS.vi"("Enum"=POST_ANALYSIS_ENUM."SAVE IMAGE", "error in"=w924, "IMAGE FILE PATH"=w923) -> ("error out"=w922:errorcluster)  [unwired: 7 in, 1 out]
                    n777 = call "Stall Data Flow.vim"("value in"=w922, "milliseconds to wait"=u32 1000) -> ("value out"=w913:errorcluster)  [unwired: 1 out]
                    n778 = local read "Test File List :"() -> (w930:string)
                    n779 = call "IMAGE ANALYSIS.vi"("Enum"=POST_ANALYSIS_ENUM."MINIMIZE UI", "error in"=w913) -> ("error out"=w920:errorcluster)  [unwired: 8 in, 1 out]
                    n780 = Bundle By Name(cluster=T25 {"File Name"="", "Test Method"="", "Operator"="", "Fuel Description"="", "Date and time"=""} ("Main Ref"), "Test Method"=w911, "File Name"=w930) -> (w931:T25)
                    n781 = call "Stall Data Flow.vim"("value in"=w920, "milliseconds to wait"=u32 1500) -> ("value out"=w915:errorcluster)  [unwired: 1 out]
                    n782 = call "duf file read.vi"("error in (no error)"=w915, "Main Ref"=w931) -> ("error out"=w929:errorcluster, "Main Ref 2"=w927:T25)  [unwired: 8 in]
                    n783 = call "DETECTION REPORT for manual.vi"("error in (no error)"=w929, "return value 3"=w926, "Image File Path"=w928, "Main Ref"=w927) -> ("error out"=w925:errorcluster)  [unwired: 7 in]
                    n784 = call <vilib>:"Clear Errors.vi"("error in (no error)"=w925) -> ("error out"=w916:errorcluster)  [unwired: 5 in, 1 out]
                    n785 = call "IMAGE ANALYSIS.vi"("Enum"=POST_ANALYSIS_ENUM."MINIMIZE UI", "error in"=w916) -> ("error out"=w918:errorcluster)  [unwired: 8 in, 1 out]
                  }
                  frame #1 {
                    n786 = local write "Main Tab"(T2."HOME" ("Main Tab")) -> ()
                    n787 = local write "Main Dashboard Buttons"(T1."Home" ("Main Dashboard Buttons")) -> ()
                  }
                }
              }
              frame "Calibrate" {
              }
            }
          }
          frame #2 {
            n788 = Not(x=w1000) -> (.not. x?=w999:bool)
            n789 = local write "Confirm Measrurement"(w999) -> ()
            n790 = local read "Calibration Tab"() -> (w998:enum32{"Measrument", "Calibrate"})
            n791 = case shown="\"Measrument\", Default" w998 {
              frame "Measrument", Default {
                (unwired) T20."HOME" ("Main Tab")
                n792 = local write "Main Tab"(T2."HOME" ("Main Tab")) -> ()
              }
              frame "Calibrate" {
              }
            }
          }
        }
      }
    }
    n793 = local read "Humidity"() -> (w743:bool)
    n794 = local read "Save Change"() -> (w748:bool)
    n795 = local read "Calibrate"() -> (w749:bool)
    n796 = local read "Auto Start Test"() -> (w744:bool)
    n797 = case shown="True" w749 {
      selector: w749 -> [_ w856]
      frame False {
      }
      frame True {
        n798 = Not(x=w856) -> (.not. x?=w855:bool)
        n799 = local write "Calibrate"(w855) -> ()
        n800 = local write "Calibration Tab"(enum32{"Measrument", "Calibrate"}."Calibrate" ("Calibration Tab")) -> ()
      }
    }
    n801 = case shown="True" w748 {
      selector: w748 -> [_ w800]
      frame False {
      }
      frame True {
        n802 = stacked-sequence {
          tunnel: w800 -> [_ _ _ _ w854]
          frame #0 {
            n803 = call "IMAGE ANALYSIS.vi"("Enum"=POST_ANALYSIS_ENUM."HIDE UI") -> ()  [unwired: 9 in, 2 out]
          }
          frame #1 {
            n804 = local read "100x gain"() -> (w802:dbl)
            n805 = local read "10x Gain"() -> (w803:dbl)
            n806 = local read "5x Gain"() -> (w804:dbl)
            n807 = Number To Fractional String(number=w803, width (-)=i16 4, precision (6)=i16 7) -> (F-format string=w825:string)  [unwired: 1 in]
            n808 = Number To Fractional String(number=0.0, width (-)=i16 4, precision (6)=i16 7) -> (F-format string=w820:string)  [unwired: 1 in]
            n809 = Number To Fractional String(number=w802, width (-)=i16 4, precision (6)=i16 7) -> (F-format string=w808:string)  [unwired: 1 in]
            n810 = Number To Fractional String(number=w804, width (-)=i16 10 ("precision (6)"), precision (6)=i16 7) -> (F-format string=w834:string)  [unwired: 1 in]
            n811 = Concatenate Strings("[CH1]" ("string"), w834, " - 5x Gain" ("string"), "\r") -> (w824:string)
            n812 = Concatenate Strings("[CH2]" ("string"), w825, " - 10x Gain" ("string"), "\r") -> (w823:string)
            n813 = Concatenate Strings("[CH3]" ("string"), w820, " - 20x Gain" ("string"), "\r") -> (w814:string)
            n814 = Concatenate Strings("[CH4]" ("string"), w808, " - 100x Gain" ("string"), "\r") -> (w807:string)
            n815 = String To Path(string="C:\\LAB-IQ\\Image Calibrate v01.dcf") -> (path=w837:path)
            n816 = Concatenate Strings(w824, w823, w814, w807) -> (w822:string)
            n817 = call <vilib>:"Write Characters To File.vi"("append to file? (new file:F)"=FALSE, "character string"=w822, "file path (dialog if empty)"=w837) -> ()  [unwired: 2 in, 1 out]
          }
          frame #2 {
            n818 = String To Path(string="C:\\LAB-IQ\\Image Calibrate v01.dcf") -> (path=w840:path)
            n819 = Open/Create/Replace File ("Open File")(file path (use dialog)=w840) -> (refnum out=w841:refnum<file>)  [unwired: 5 in, 2 out]
            n820 = for {
              N: 4 -> [_]
              tunnel: w841 -> [w847]
              i -> [w843]
              n821 = Read from Text File ("Read File")(file (use dialog)=w847) -> (text=w848:string)  [unwired: 3 in, 3 out]
              n822 = String Subset(string=w848, offset (0)=6, length (rest)=10 ("length (rest)")) -> (substring=w844:string)
              n823 = Fract/Exp String To Number(string=w844) -> (number=w842:dbl)  [unwired: 3 in, 1 out]
              n824 = case shown="3" w843 {
                tunnel: w842 -> [w849 w850 _ w851 _]
                frame 0 {
                  n825 = local write "5x Gain"(w849) -> ()
                }
                frame 1 {
                  n826 = local write "10x Gain"(w850) -> ()
                }
                frame 2 {
                }
                frame 3 {
                  n827 = local write "100x gain"(w851) -> ()
                }
                frame 4, Default {
                }
              }
            }
          }
          frame #3 {
            n828 = call "IMAGE ANALYSIS.vi"("Enum"=POST_ANALYSIS_ENUM."SHOW UI") -> ()  [unwired: 9 in, 2 out]
          }
          frame #4 {
            n829 = Not(x=w854) -> (.not. x?=w853:bool)
            n830 = local write "Save Change"(w853) -> ()
          }
        }
      }
    }
    n831 = case shown="False" w744 {
      tunnel: w743 -> [w770 _]
      frame False {
        n832 = case shown="True" w770 {
          frame False {
          }
          frame True {
            n833 = local read "Set Humidity:"() -> (w774:dbl)
            n834 = local read "Set Humidity:"() -> (w777:dbl)
            n835 = local read "Humidity ( %RH )"() -> (w778:dbl)
            n836 = Subtract(x=w774, y=2.0) -> (x-y=w772:dbl)
            n837 = Add(x=w777, y=2.0) -> (x+y=w773:dbl)
            n838 = In Range and Coerce(upper limit=w773, x=w778, lower limit=w772) -> (In Range?=w771:bool)  [unwired: 1 out]
            n839 = case shown="True" w771 {
              frame False {
              }
              frame True {
                n840 = case shown="True" "Manual Humididty Reached" {
                  selector: "Manual Humididty Reached" -> [_ w781]
                  frame False {
                  }
                  frame True {
                    n841 = Not(x=w781) -> (.not. x?=w780:bool)
                    n842 = local write "Manual Humididty Reached"(w780) -> ()
                    n843 = local read "EVENT LOG"() -> (w783:string)
                    n844 = call "Event Log.vi"("Content"="Target Humidity reached", "EVENT LOG"=w783) -> ("EVENT LOG"=w782:string)  [unwired: 8 in, 1 out]
                    n845 = local write "EVENT LOG"(w782) -> ()
                  }
                }
              }
            }
          }
        }
      }
      frame True {
        n846 = local write "Manual Humididty Reached"(TRUE ("Manual Humididty Reached")) -> ()
      }
    }
    n847 = local read "Cap Live Image"() -> (w764:bool)
    n848 = local read "SCAR MEASURMENT"() -> (w767:enum32{"Auto Scar", "Manual Scar"})
    n849 = Wait (ms)(milliseconds to wait=u32 250) -> ()  [unwired: 1 out]
    n850 = Equal?(x=w767, y=enum32{"Auto Scar", "Manual Scar"}."Manual Scar" ("SCAR MEASURMENT")) -> (x = y?=w765:bool)
    n851 = And(x=w765, y=w764) -> (x .and. y?=w763:bool)
    n852 = case shown="True" w763 {
      selector: w763 -> [_ w1079]
      frame False {
      }
      frame True {
        n853 = stacked-sequence {
          tunnel: [_ _ _ w1094 _] -> _
          tunnel: w1079 -> [_ _ _ _ w1101]
          frame #0 {
            w1080 = 0.0
            n854 = local write "Major Axis"(w1080) -> ()
            n855 = local write "Minor Axis"(w1080) -> ()
            n856 = local write "Average"(w1080) -> ()
          }
          frame #1 {
            n857 = call "CAMERA LIVE FEED FGV.vi"("Enum - Menu"=CAMERA_LIVE_FEED_ENUM."CAMERA MINIMIZE") -> ()  [unwired: 9 in, 2 out]
          }
          frame #2 {
            n858 = local read "FILE 3"() -> (w1088:string)
            n859 = call <vilib>:"Trim Whitespace.vi"("string"="C:\\LAB-IQ\\images\\") -> ("trimmed string"=w1090:string)  [unwired: 1 in]
            n860 = String To Path(string=w1090) -> (path=w1089:path)
            n861 = Concatenate Strings(w1088, ".png" ("string")) -> (w1087:string)
            n862 = Build Path(base path=w1089, name or relative path=w1087) -> (appended path=w1085:path)
            n863 = Path To String(path=w1085) -> (string=w1084:string)
            n864 = call "CAMERA LIVE FEED FGV.vi"("Enum - Menu"=CAMERA_LIVE_FEED_ENUM."CAMERA SAVE", "Image Path"=w1084) -> ("error out"=w1082:errorcluster)  [unwired: 8 in, 1 out]
            n865 = case shown="No Error" w1082 {
              frame No Error {
                n866 = One Button Dialog(message="Image saved successfully") -> ()  [unwired: 1 in, 1 out]
              }
              frame Error {
              }
            }
          }
          frame #3 {
            n867 = call "LIST FILE NAMES.vi"() -> ("error out"=w1096:errorcluster, "filenames"=w1093:string[])  [unwired: 10 in]
            n868 = call "IMAGE ANALYSIS.vi"("Enum"=POST_ANALYSIS_ENUM."SHOW UI", "error in"=w1096) -> ("error out"=w1094:errorcluster)  [unwired: 8 in, 1 out]
            n869 = property on="Test File List :" class="CmbBox"("Strings[]"=w1093) -> ()  [unwired: 2 in, 2 out]
          }
          frame #4 {
            (unwired) T24."Report" ("Main Dashboard Buttons")
            (unwired) T26."Report" ("Main Dashboard Buttons")
            n870 = Not(x=w1101) -> (.not. x?=w1100:bool)
            n871 = local write "Zoom Factore"(0.0 ("Zoom Factore")) -> ()
            n872 = local write "Cap Live Image"(w1100) -> ()
            n873 = local write "Main Tab"(T2."Adv Scar Report" ("Main Tab")) -> ()
            n874 = property on="Cap Live Image" class="Bool (strict)"("BoolText.Text"="Capture Image" ("Boolean Text.Text")) -> ()  [unwired: 2 in, 2 out]
            n875 = local write "Main Dashboard Buttons"(T1."Report" ("Main Dashboard Buttons")) -> ()
          }
        }
      }
    }
    n876 = local read "change Gain"() -> (w747:bool)
    n877 = local read "Back Square"() -> (w746:bool)
    n878 = case shown="True" w747 {
      selector: w747 -> [_ w791]
      frame False {
      }
      frame True {
        n879 = stacked-sequence {
          tunnel: w791 -> [_ w799]
          frame #0 {
            n880 = local read "Actual (µm)"() -> (w795:dbl)
            n881 = local read "Pixel Value"() -> (w794:dbl)
            n882 = local read "Magnification :"() -> (w793:string)
            n883 = Divide(x=w795, y=w794) -> (x/y=w792:dbl)
            n884 = case shown="\"10x\"" w793 {
              tunnel: w792 -> [w796 w797]
              frame "10x" {
                n885 = local write "10x Gain"(w796) -> ()
              }
              frame "5x", Default {
                n886 = local write "5x Gain"(w797) -> ()
              }
            }
          }
          frame #1 {
            n887 = Not(x=w799) -> (.not. x?=w798:bool)
            n888 = local write "change Gain"(w798) -> ()
          }
        }
      }
    }
    n889 = case shown="True" w746 {
      selector: w746 -> [_ w789]
      frame False {
      }
      frame True {
        n890 = Not(x=w789) -> (.not. x?=w788:bool)
        n891 = local write "Back Square"(w788) -> ()
        n892 = local write "Calibration Tab"(enum32{"Measrument", "Calibrate"}."Measrument" ("Calibration Tab")) -> ()
      }
    }
    n893 = local read "Rectangle Tool"() -> (w758:bool)
    n894 = local read "Clear ROI Tool"() -> (w757:bool)
    n895 = local read "Open Image"() -> (w762:bool)
    n896 = local read "line tool"() -> (w759:bool)
    n897 = local read "OUT"() -> (w760:bool)
    n898 = local read "In"() -> (w761:bool)
    n899 = case shown="True" w762 {
      selector: w762 -> [_ w1067]
      tunnel: [w1063 w1069] -> _
      tunnel: w752 -> [w1063 w1068]
      frame False {
      }
      frame True {
        n900 = Not(x=w1067) -> (.not. x?=w1066:bool)
        n901 = local write "Open Image"(w1066) -> ()
        n902 = call "IMAGE ANALYSIS.vi"("Enum"=POST_ANALYSIS_ENUM."HIDE UI", "error in"=w1068) -> ("error out"=w1076:errorcluster)  [unwired: 8 in, 1 out]
        n903 = call "File Dialog"("start path"=path "C:/LAB-IQ/images", "error in"=w1076) -> ("selected path"=w1065:path, "error out"=w1074:errorcluster)  [unwired: 10 in, 2 out]
        "Image path  2" <- w1065
        n904 = call <vilib>:"Clear Errors.vi"("error in (no error)"=w1074) -> ("error out"=w1073:errorcluster)  [unwired: 5 in, 1 out]
        n905 = call "IMAGE ANALYSIS.vi"("Enum"=POST_ANALYSIS_ENUM."OPEN FILE", "error in"=w1073, "File Path"=w1065) -> ("error out"=w1072:errorcluster)  [unwired: 7 in, 1 out]
        n906 = call <vilib>:"Clear Errors.vi"("error in (no error)"=w1072) -> ("error out"=w1071:errorcluster)  [unwired: 5 in, 1 out]
